vi "StepRealtime_IP7.vi"() -> ()   [LabVIEW 2014]
doc: "This VI was generated automatically using the FPGA Wizard. You can modify the VI normally."
uses:
  <vilib>/Platform/TimedLoop/XDataNode/timing_clust.ctl
  <vilib>/Platform/TimedLoop/XDataNode/nitl_modes.ctl
  <vilib>/Platform/TimedLoop/XDataNode/wakeup.ctl
  <vilib>/FPGAPlugInAG/sbRIO-9642/niLvFpga_Open_sbRIO-9642.vi
  <vilib>/rvi/interface/common/dynamic/niFpgaDynamicAddResources.vi
  <vilib>/FPGAPlugInAG/Dynamic/niLvFpga_Reset_Dynamic.vi
  <vilib>/FPGAPlugInAG/Dynamic/niLvFpga_Run_Dynamic.vi
  <vilib>/Utility/error.llb/Error Cluster From Error Code.vi
  <vilib>/rvi/errors/niLvFpgaAdjustHostInterfaceError.vi
  <vilib>/FPGAPlugInAG/Dynamic/niLvFpga_Close_Dynamic.vi
  <vilib>/rvi/interface/nirviOpenFPGA/nirviOpenFPGA.xnode
  FPGA Bitfiles/PPDControlLab3_FPGA_IP7.lvbitx
  <vilib>/rvi/interface/nirviMethod/nirviMethod.xnode
  <vilib>/Platform/TimedLoop/XDataNode/XDataNode.xnode
  <vilib>/rvi/interface/nirviReadWriteControl/nirviReadWriteControl.xnode
  <vilib>/rvi/interface/nirviCloseFPGA/nirviCloseFPGA.xnode
  SysIDRealtime.lvlib
  <vilib>/rvi/interface/Simulation/niFpgaSimulationCallBeginRW.vi
  <vilib>/Platform/TimedLoop/XDataNode/XDNodeRunTimeDep.lvlib
  NiFpgaLv.dll
panel:
  out "Ratio":fxp<+/-,32,7>
  in  "Gain":fxp<+/-,32,7>=0.006999999284744263
  in  "Radio Buttons":enum32{"Radio Selection 1", "Radio Selection 2"}(radio)
  in  "OK Button":bool
  out "Step Response":dynamicdata(graph)=[{"t0"=timestamp(0 s since 1904-01-01), "dt"=1.0, "Y"=array[2048 elements]}, {"t0"=timestamp(0 s since 1904-01-01), "dt"=1.0, "Y"=array[2048 elements]}, {"t0"=timestamp(0 s since 1904-01-01), "dt"=1.0, "Y"=array[2048 elements]}]
  in  "samples":i32=2048
  in  "Reference":i32
  in  "Quad Reset":bool=TRUE
  in  "DGain":fxp<+/-,32,7>
  in  "PGain":fxp<+/-,32,7>
  out "Amp In":dbl[](graph)
  out "Amp Cpmmand":fxp<+/-,20,5>
  out "Iteration Duration":i64
  out "Position":i32[](graph)
  in  "Control Rate (ticks)":u32=10000
  in  "Period (us)":i64=1000
  out "Finished Late? [i-1]":bool
  out "quad saved (Port0/DIO0,Port0/DIO1)":cluster{"Position":i32, "Index Count":u16}
  out "quad pos (Port0/DIO0,Port0/DIO1)":i32
  out "Late? Latched":bool
  in  "Local Stop 0":bool
  in  "Start 0":bool
  in  "Loop Rate (Hz)":dbl=100000.0
  out "Calculated Rate (Hz)":dbl
  out "error out":errorcluster
  in  "Global Stop":bool
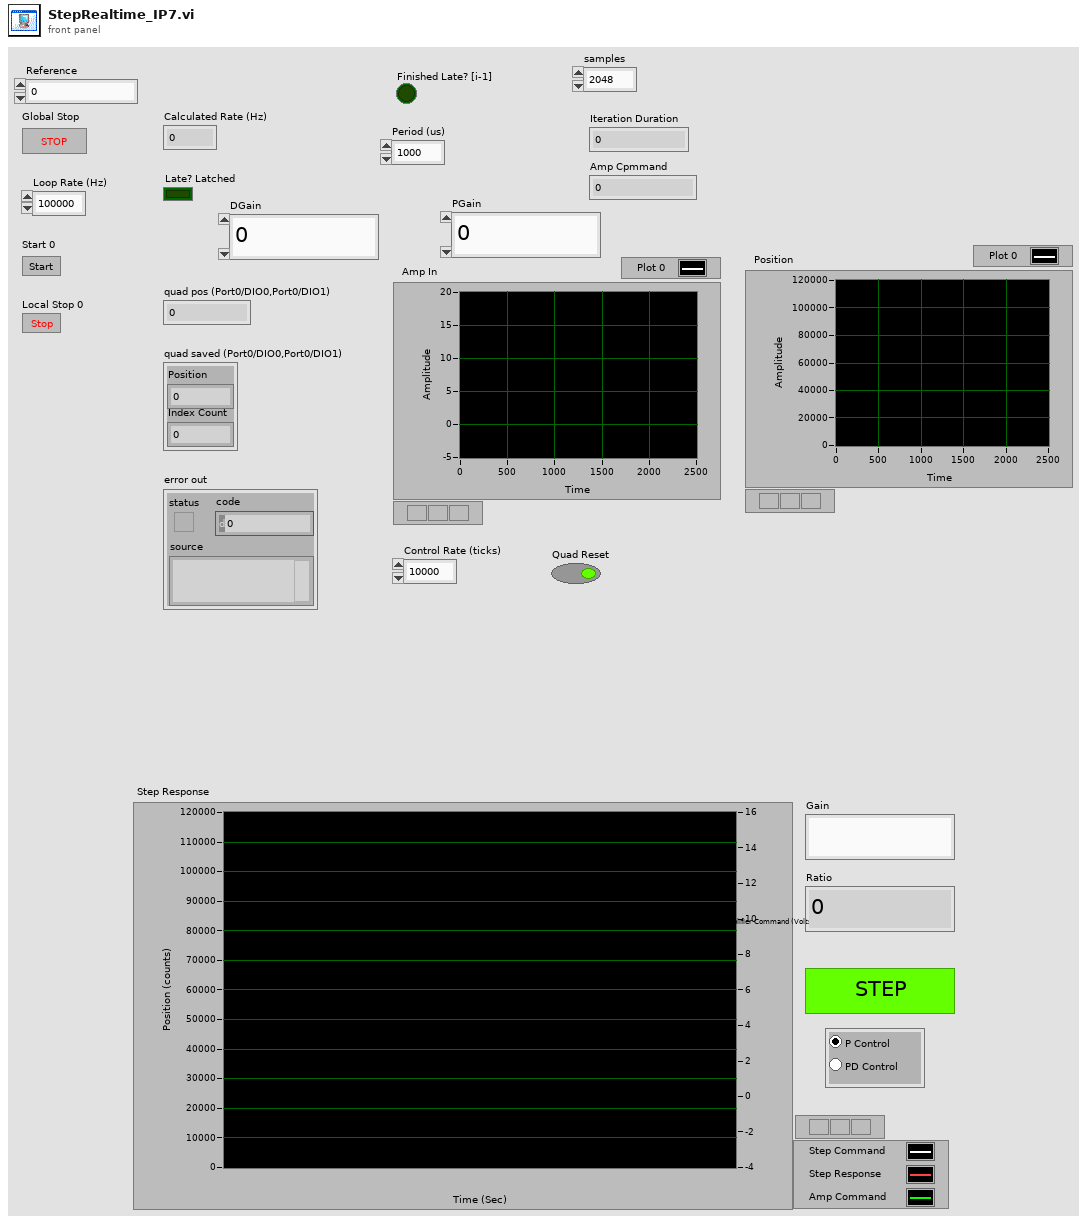
[diagram p1: front panel]
types:
  T1 = typedef "XDNodeRunTimeDep.lvlib/timing_clust.ctl" = cluster{"Expected End [f-1]":u64, "Actual End [f-1]":u64, "Finished Late? [f-1]":bool, "Expected End [i-1]":u64, "Actual End [i-1]":u64, "Finished Late? [i-1]":bool, "Expected Start [i]":u64, "Actual Start [i]":u64, "Expected Start [f]":u64, "Actual Start [f]":u64, "Source Name":string, "Structure Name":string, "Period":i64, "Deadline":i64, "Offset":i64, "Start":i64, "Priority":i32, "Timeout":i32, "Mode":T2, "Wakeup Reason":T3, "Error":errorcluster, "Source Type":string, "Secondary Source Type":string, "Global End Time":u64, "Global Start Time":u64, "Frame Duration":u64, "Iteration Duration":u64, "Assigned CPU":i32, "I/O Scan Engine Mode":u32}
  T2 = typedef "XDNodeRunTimeDep.lvlib/nitl_modes.ctl" = enum32{"No Change", "Process missed periods, maintain original phase", "Discard missed periods, maintain original phase", "Process missed periods, ignore original phase", "Discard missed periods, ignore original phase"}
  T3 = typedef "XDNodeRunTimeDep.lvlib/wakeup.ctl" = enum32{"Normal", "Aborted", "Asynchronous wakeup", "Timing source error", "Timed loop error", "Timeout"}
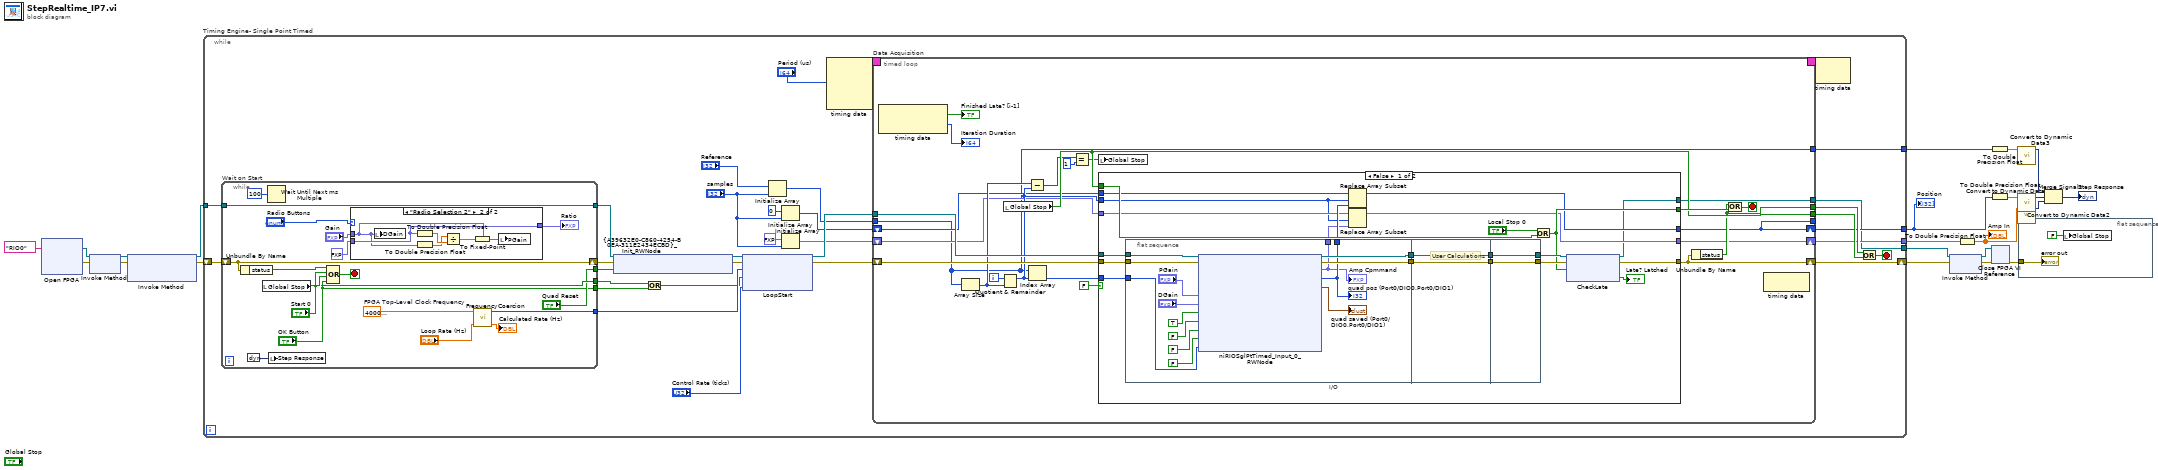
[diagram p0: block diagram]
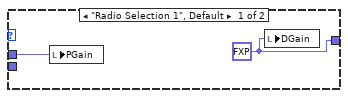
[diagram p3: hidden frame]
diagram:
  n1 = xnode ("Open FPGA")("resource name"=tag "RIO0") -> ("FPGA VI Reference Out"=w18:refnum<k20>, "error out"=w19:errorcluster)  [unwired: 1 in]
  n2 = xnode ("Invoke Method")("FPGA VI Reference In"=w18, "error in"=w19) -> ("FPGA VI Reference Out"=w21:refnum<k20>, "error out"=w22:errorcluster)
  n3 = xnode ("Invoke Method")("FPGA VI Reference In"=w21, "error in"=w22) -> ("FPGA VI Reference Out"=w5:refnum<k20>, "error out"=w20:errorcluster)  [unwired: 1 in]
  n4 = while "Timing Engine- Single Point Timed" {
    tunnel: w5 -> [w51]
    shift-right: [w50] -> w3
    shift-left: w20 -> [w54]
    tunnel: [w32] -> w11
    tunnel: [w33] -> w16
    tunnel: [w27] -> w9
    tunnel: [w23] -> w4
    stop <- w45 stop-if-true
    n5 = while "Wait on Start" {
      tunnel: w51 -> [w145]
      tunnel: [w145] -> w49
      tunnel: [w137] -> w42
      tunnel: ["Start 0"] -> w26
      shift-right: [w139] -> w48
      shift-left: w54 -> [w139]
      tunnel: ["Quad Reset"] -> w31
      tunnel: ["OK Button"] -> w25
      stop <- w146 stop-if-true
      w140 = 40000000.0  # FPGA Top-Level Clock Frequency
      n6 = Unbundle By Name(w139) -> ("status"=w138:bool)
      n7 = local read "Global Stop"() -> (w143:bool)
      n8 = Wait Until Next ms Multiple(millisecond multiple=u32 100) -> ()  [unwired: 1 out]
      n9 = local write "Step Response"(dynamicdata [] ("Step Response")) -> ()
      n10 = Compound Arithmetic op=OR(w138, "Start 0", w143, "OK Button") -> (w146:bool)
      n11 = case shown="\"Radio Selection 2\"" "Radio Buttons" {
        tunnel: "Gain" -> [w148 w149]
        tunnel: fxp<+/-,32,7> 40.0 ("Ratio") -> [_ w150]
        tunnel: [w147 w150] -> w130
        frame "Radio Selection 1", Default {
          w147 = fxp<+/-,32,7> 0.0 ("DGain")
          n12 = local write "PGain"(w148) -> ()
          n13 = local write "DGain"(w147) -> ()
        }
        frame "Radio Selection 2" {
          n14 = local write "DGain"(w149) -> ()
          n15 = To Double Precision Float(number=w150) -> (double precision float=w154:dbl)
          n16 = To Double Precision Float(number=w149) -> (double precision float=w153:dbl)
          n17 = Divide(x=w153, y=w154) -> (x/y=w152:dbl)
          n18 = To Fixed-Point(fixed-point type=w149, number=w152) -> (fixed-point=w151:fxp<+/-,32,7>)
          n19 = local write "PGain"(w151) -> ()
        }
      }
      "Ratio" <- w130
      n20 = call "FrequencyCoercion.vi"("Loop Rate (Hz)"="Loop Rate (Hz)", "FPGA Top-Level Clock Frequency"=w140) -> ("Actual Rate (Hz)"=→"Calculated Rate (Hz)":dbl, "FPGA Ticks"=w137:u32)  [unwired: 2 in]
    }
    n21 = xnode ("{A39632E0-C860-4254-B0EA-311E2434ECBD}_Init_RWNode")("FPGA VI Reference In"=w49, "error in"=w48, "quad reset (Port0/DIO0,Port0/DIO1)"=w31) -> ("FPGA VI Reference Out"=w43:refnum<k20>, "error out"=w47:errorcluster)
    n22 = Or(x=w26, y=w25) -> (x .or. y?=w24:bool)
    n23 = xnode ("LoopStart")("FPGA VI Reference In"=w43, "error in"=w47, "Loop Rate (Ticks)"=w42, "Start 0"=w24, "Control Rate (ticks)"="Control Rate (ticks)") -> ("FPGA VI Reference Out"=w53:refnum<k20>, "error out"=w52:errorcluster)
    n24 = Initialize Array("Reference", "samples") -> (w28:i32[])
    n25 = Initialize Array(0 ("quad pos (Port0/DIO0,Port0/DIO1)"), "samples") -> (w36:i32[])
    n26 = Initialize Array(fxp<+/-,20,5> 0.0 ("Amp Cpmmand"), "samples") -> (w34:fxp<+/-,20,5>[])
    n27 = node-c288("Period (us)") -> (w41:T1)  [unwired: 3 in]
    n28 = timed-loop "Data Acquisition" {
      tunnel: w53 -> [w72]
      tunnel: [w74] -> w46
      tunnel: [w73] -> w44
      shift-right: [w77] -> w50
      shift-left: w52 -> [w71]
      timing: w41 -> [_]
      timing-out: [_] -> w40
      tunnel: w28 -> [w56]
      tunnel: [w58] -> _
      shift-right: [w57] -> w33
      shift-left: w34 -> [w59]
      shift-right: [w58] -> w32
      shift-left: w36 -> [w61]
      tunnel: [w56] -> w27
      tunnel: [w55] -> w23
      i -> [w68]
      stop <- w75 stop-if-true
      n29 = node-c288() -> (→"Finished Late? [i-1]":bool, →"Iteration Duration":i64)  [unwired: 1 in]
      n30 = Array Size(array=w56) -> (size(s)=w66:i32)
      n31 = Quotient & Remainder(x=w68, y=w66) -> (x-y*floor(x/y)=w62:i32)  [unwired: 1 out]
      n32 = local read "Global Stop"() -> (w74:bool)
      n33 = Subtract(x=w66, y=w62) -> (x-y=w65:i32)
      n34 = Index Array(array=w56, index=w62) -> (element=w67:i32)
      n35 = Equal?(x=w65, y=1) -> (x = y?=w63:bool)
      n36 = local write "Global Stop"(w63) -> ()
      n37 = case "Timeout" shown="False" FALSE {
        tunnel: w72 -> [w98 w122]
        tunnel: w71 -> [w97 w124]
        tunnel: [w91 w124] -> w77
        tunnel: [w93 w123] -> w76
        tunnel: w74 -> [w94 w123]
        tunnel: w67 -> [w83 _]
        tunnel: w62 -> [w85 _]
        tunnel: w61 -> [w89 _]
        tunnel: [w88 _] -> w58
        tunnel: w59 -> [w87 _]
        tunnel: [w84 _] -> w57
        tunnel: [w82 w122] -> w55
        frame False {
          n38 = flat-sequence "I/O" {
            tunnel: w98 -> [w115]
            tunnel: w97 -> [w117]
            tunnel: [w116] -> w103
            tunnel: [w114] -> w100
            tunnel: [w112] -> w90
            tunnel: [w111] -> w86
            tunnel: w83 -> [w104]
            tunnel: [w119] -> w102
            tunnel: w103 -> [w118]
            tunnel: w100 -> [w119]
            tunnel: [w118] -> w101
            tunnel: [w120] -> w96
            tunnel: [w121] -> w99
            tunnel: w102 -> [w121]
            tunnel: w101 -> [w120]
            frame #0 {
              n39 = xnode ("niRIOSglPtTimed_Input_0_RWNode")("FPGA VI Reference In"=w115, "error in"=w117, "PGain"="PGain", "DGain"="DGain", "Amp Enable"=TRUE, "Amp Reset"=FALSE, "Brake"=FALSE, "quad reset (Port0/DIO0,Port0/DIO1)"=FALSE, "Reference"=w104) -> ("FPGA VI Reference Out"=w114:refnum<k20>, "error out"=w116:errorcluster, "Amp Cpmmand"=w111:fxp<+/-,20,5>, "quad pos (Port0/DIO0,Port0/DIO1)"=w112:i32, "quad saved (Port0/DIO0,Port0/DIO1)"=→"quad saved (Port0/DIO0,Port0/DIO1)":cluster{"Position":i32, "Index Count":u16})
              "quad pos (Port0/DIO0,Port0/DIO1)" <- w112
              "Amp Cpmmand" <- w111
            }
            frame #1 {
              # "User Calculations"
            }
            frame #2 {
            }
          }
          n40 = Replace Array Subset(array=w89, new element=w90, index=w85) -> (w88:i32[])
          n41 = Replace Array Subset(array=w87, new element=w86, index=w85) -> (w84:fxp<+/-,20,5>[])
          n42 = Or(x="Local Stop 0", y=w94) -> (x .or. y?=w93:bool)
          n43 = xnode ("CheckLate")("FPGA VI Reference In"=w99, "error in"=w96, "Local Stop 0"=w93) -> ("FPGA VI Reference Out"=w82:refnum<k20>, "error out"=w91:errorcluster, "Late? Latched"=→"Late? Latched":bool)
        }
        frame True {
          # "Timeout waiting for an interrupt. This case checks the state of the global stop.\nIf global stop is not set, then loop around to wait for an interrupt again."
        }
      }
      n44 = Unbundle By Name(w77) -> ("status"=w73:bool)
      n45 = Or(x=w73, y=w76) -> (x .or. y?=w75:bool)
      n46 = node-c288() -> ()  [unwired: 1 in, 1 out]
    }
    n47 = node-c288(w40) -> ()  [unwired: 1 out]
    n48 = Or(x=w44, y=w46) -> (x .or. y?=w45:bool)
  }
  "Position" <- w11
  n49 = xnode "Invoke Method"("FPGA VI Reference In"=w4, "error in"=w3) -> ("FPGA VI Reference Out"=w2:refnum<k20>, "error out"=w1:errorcluster)
  n50 = To Double Precision Float(number=w16) -> (double precision float=w13:dbl[])
  "Amp In" <- w13
  n51 = To Double Precision Float(number=w9) -> (double precision float=w8:dbl[])
  n52 = To Double Precision Float(number=w11) -> (double precision float=w10:dbl[])
  n53 = xnode ("Close FPGA VI Reference")("FPGA VI Reference In"=w2, "error in"=w1) -> ("error out"=w17:errorcluster)
  n54 = call "Convert to Dynamic Data3"("Array"=w8) -> ("Dynamic Data Type"=w7:dynamicdata)  [unwired: 3 in]
  n55 = call "Convert to Dynamic Data"("Array"=w10) -> ("Dynamic Data Type"=w14:dynamicdata)  [unwired: 3 in]
  n56 = call "Convert to Dynamic Data2"("Array"=w13) -> ("Dynamic Data Type"=w12:dynamicdata)  [unwired: 3 in]
  n57 = flat-sequence {
    tunnel: w17 -> [w156]
    frame #0 {
      n58 = local write "Global Stop"(FALSE ("Global Stop")) -> ()
      "error out" <- w156
    }
  }
  n59 = Merge Signals(w7, w14, w12) -> (→"Step Response":dynamicdata)
